vi "Reposition Single Wheel on Steering Frame.vi"(5 "x position":dbl, 6 "frame angle (rad)":dbl=nan, 7 "y position":dbl, 8 "error in (no error)":errorcluster, 10 "wheel index":i32, 11 "steering frame in":refnum<class "NI_Robotics_Steering Frame.lvclass">) -> (0 "error out":errorcluster, 1 "found?":bool, 3 "steering frame out":refnum<class "NI_Robotics_Steering Frame.lvclass">)   [LabVIEW 2017, in "NI_Robotics_Steering Frame.lvclass"]
doc: "Changes the location of the wheel or wheels to the position and angle you specify. You must manually select the polymorphic instance to use."
uses:
  <vilib>/robotics/Steering/Steering Frame/NI_Robotics_Steering Frame.lvclass
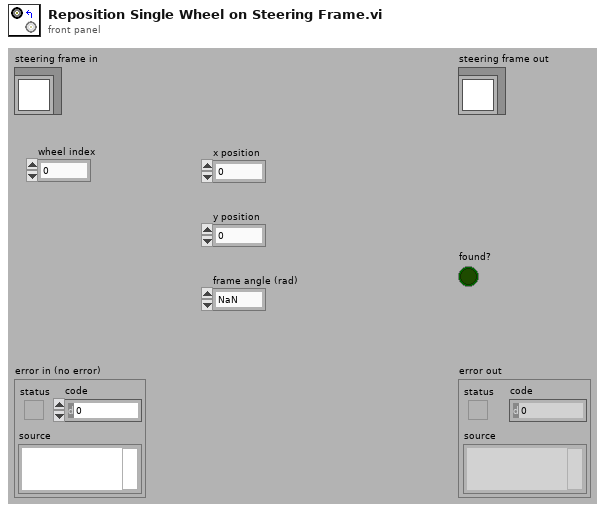
[diagram p1: front panel]
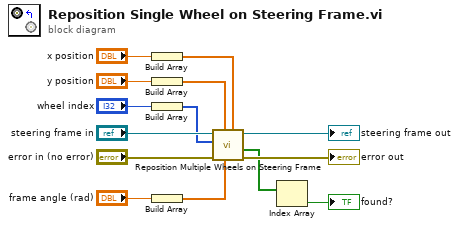
[diagram p0: block diagram]
diagram:
  n1 = Build Array("x position") -> (w9:dbl[])
  n2 = Build Array("y position") -> (w7:dbl[])
  n3 = Build Array("wheel index") -> (w5:i32[])
  n4 = Build Array("frame angle (rad)") -> (w3:dbl[])
  n5 = call <vilib>:"Reposition Multiple Wheels on Steering Frame.vi"("x positions"=w9, "frame angles (rad)"=w3, "y positions"=w7, "error in (no error)"="error in (no error)", "wheel indexes"=w5, "steering frame in"="steering frame in") -> ("error out"=→"error out":errorcluster, "found?"=w2:bool[], "steering frame out"=→"steering frame out":refnum<class "NI_Robotics_Steering Frame.lvclass">)  [unwired: 3 in]
  n6 = Index Array(array=w2) -> (element=→"found?":bool)  [unwired: 1 in]
